vi "RobotDrive.vi"   [LabVIEW 2013]
uses:
  Robot Global Data.vi
  <vilib>/Rock Robotics/WPI/RobotDrive/WPI_RobotDriveArcadeDrive_Standard(NoSaturation).vi
  <vilib>/Rock Robotics/WPI/RobotDrive/WPI_RobotDriveGetSetRefNum.vi
types:
  T1 = cluster{"J1 Y Axis":dbl, "J2 Y Axis":dbl, "J3 Y Axis":dbl, "J3 Throttle":dbl}
  T2 = cluster{"Activate Elevator":bool, "Shoot":bool, "Bridge Direction":bool, "Low Speed":bool, "Med Speed":bool, "High Speed":bool, "Loader Down":bool, "Activate Bridge":bool, "Limit Shooter":bool, "Elevator Down":bool, "Reverse":bool, "Vision Processing":bool}
  T3 = typedef "WPI_RobotDriveDevRef.ctl" = cluster{"DevStatus":errorcluster, "Motors[]":T4[], "Square Inputs":bool, "Max Output":dbl, "Isochronous":bool}
  T4 = typedef "WPI_MotorControlDeviceRef.ctl" = cluster{"DeviceStatus":errorcluster, "Type":enum16{"PWM", "CAN"}, "PWM":cluster{"Digital Module":T5, "PWM Channel":T6, "DeadBand":T7}, "CAN":cluster{"Device Number":u8, "Control Mode":T8, "Semaphore":T9, "Max Vout":dbl}, "Invert":bool, "TransformRef":T10, "InvTransformRef":T10}
  T5 = typedef "FPGA_TypedefDigitalModule.ctl" = enum16{"Digital Module 1", "Digital Module 2"}
  T6 = typedef "FPGA_DIOPWMChannel.ctl" = enum8{"PWM 1", "PWM 2", "PWM 3", "PWM 4", "PWM 5", "PWM 6", "PWM 7", "PWM 8", "PWM 9", "PWM 10", "Invalid"}
  T7 = typedef "WPI_PWMDeadband.ctl" = cluster{"Name":string, "maxPositivePwm":i32, "minPositivePwm":i32, "centerPwm":i32, "maxNegativePwm":i32, "minNegativePwm":i32, "angularRange":u16}
  T8 = typedef "WPI_CANJaguar_ControlMode.ctl" = enum8{"Percent VBus", "Current", "Speed", "Position", "Voltage"}
  T9 = typedef "Semaphore RefNum" = refnum<k1>
  T10 = typedef "WPI_PWMTransform_ConPane.ctl" = refnum<vi>
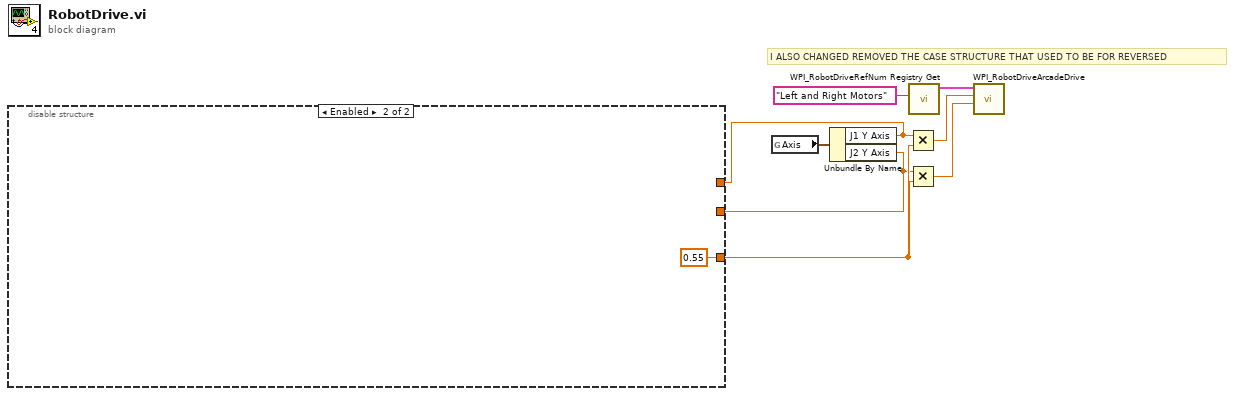
[diagram p0: block diagram]
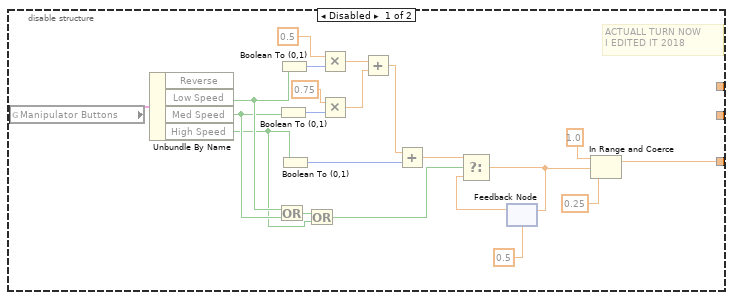
[diagram p2: hidden frame]
diagram:
  # "I ALSO CHANGED REMOVED THE CASE STRUCTURE THAT USED TO BE FOR REVERSED"
  n1 = global read "Robot Global Data.vi" "Axis"() -> (w3:T1)
  n2 = Unbundle By Name(w3) -> ("J1 Y Axis"=w2:dbl, "J2 Y Axis"=w1:dbl)
  n3 = disable-structure shown="Enabled" {
    disable-tunnel: w1 -> [_ _]
    disable-tunnel: w2 -> [_ _]
    disable-tunnel: [w10 0.55 ("upper limit")] -> w8
    frame Disabled {
      # "ACTUALL TURN NOW\nI EDITED IT 2018"
      n4 = global read "Robot Global Data.vi" "Manipulator Buttons"() -> (w29:T2)
      n5 = Unbundle By Name(w29) -> ("Low Speed"=w17:bool, "Med Speed"=w16:bool, "High Speed"=w14:bool)  [unwired: 1 out]
      n6 = Or(x=w17, y=w16) -> (x .or. y?=w15:bool)
      n7 = Boolean To (0,1)(Boolean=w16) -> (0, 1=w25:i16)
      n8 = Boolean To (0,1)(Boolean=w17) -> (0, 1=w28:i16)
      n9 = Boolean To (0,1)(Boolean=w14) -> (0, 1=w21:i16)
      n10 = Or(x=w15, y=w14) -> (x .or. y?=w13:bool)
      n11 = Multiply(x=0.5, y=w28) -> (x*y=w24:dbl)
      n12 = Multiply(x=0.75, y=w25) -> (x*y=w23:dbl)
      n13 = Add(x=w24, y=w23) -> (x+y=w22:dbl)
      n14 = Add(x=w22, y=w21) -> (x+y=w18:dbl)
      n15 = feedback #1(0.5) -> (w19:dbl)
      n16 = Select(t=w18, s=w13, f=w19) -> (s? t:f=w9:dbl)
      n17 = feedback-in #1(w9) -> ()
      n18 = In Range and Coerce(upper limit=1.0, x=w9, lower limit=0.25) -> (coerced(x)=w10:dbl)  [unwired: 1 out]
    }
    frame Enabled {
    }
  }
  n19 = Multiply(x=w2, y=w8) -> (x*y=w4:dbl)
  n20 = Multiply(x=w1, y=w8) -> (x*y=w5:dbl)
  n21 = call <vilib>:"WPI_RobotDriveRefNum Registry Get.vi"("refnum name"="Left and Right Motors") -> ("RobotDriveDevRef"=w6:T3)  [unwired: 9 in, 1 out]
  n22 = call-poly <vilib>:"WPI_RobotDriveArcadeDrive.vi"("Y axis value"=w5, "X axis value"=w4, "RobotDriveDevRef"=w6) -> ()  [unwired: 6 in, 3 out]
